vi "QMdiSubWindow.vi"(5 "parent":refnum<class "QWidget.lvclass">, 8 "Error In":errorcluster, 11 "Post-Bundled Subclass":refnum<class "QMdiSubWindow.lvclass">) -> (0 "Error Out":errorcluster, 3 "New QMdiSubWindow":refnum<class "QMdiSubWindow.lvclass">)   [LabVIEW 2014, in "QMdiSubWindow.lvclass"]
doc: "LabVIEW-specific documentation is not yet available. See <b>https://doc.qt.io/qt-5/qmdisubwindow.html#QMdiSubWindow</b>"
uses:
  QMdiSubWindow.lvclass
  QWidget/QWidget.lvclass
  LQ Core/LQCoreEngine/_Internal/LQIdentity Registry Action.ctl
  LQ Core/LQIdentity/LQIdentity.lvclass/LQIdentity.ctl
  LQ Core/LQCoreEngine/LQCoreEngine.lvclass
  LQ Core/LQ Core.lvlib
  LQ Core/LQIdentity/LQIdentity.lvclass
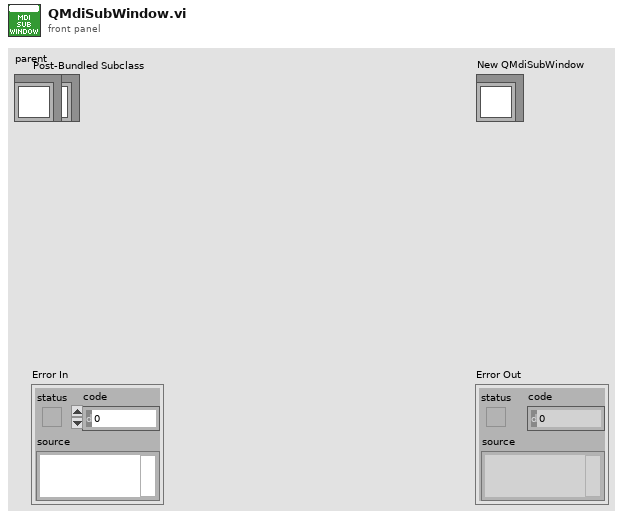
[diagram p1: front panel]
types:
  T1 = typedef "LQ Core.lvlib/LQCoreEngine.lvclass/LQIdentity Registry Action.ctl" = enum16{"Init", "Register LQIdentity", "Get LQIdentity Info", "Deregister LQIdentity"}
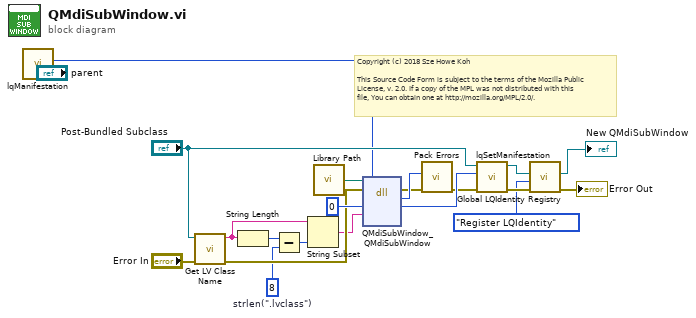
[diagram p0: block diagram]
diagram:
  w6 = 8  # strlen(".lvclass")
  # "Copyright (c) 2018 Sze Howe Koh\n\nThis Source Code Form is subject to the terms of the Mozilla Public\nLicense, v. 2.0. If a copy of the MPL was not distributed with this\nfile, You can obtain one at http://mozilla.org/MPL/2.0/."
  n1 = call "lqManifestation.vi"("LQIdentity in"="parent") -> ("Manifestation"=w1:u64)  [unwired: 9 in, 1 out]
  n2 = call <vilib>:"Get LV Class Name.vi"("error in (no error)"="Error In", "object"="Post-Bundled Subclass") -> ("error out"=w8:errorcluster, "class name"=w4:string)  [unwired: 8 in]
  n3 = String Length(string=w4) -> (length=w7:i32)
  n4 = Subtract(x=w7, y=w6) -> (x-y=w5:i32)
  n5 = String Subset(string=w4, length (rest)=w5) -> (substring=w3:string)  [unwired: 1 in]
  n6 = call "Library Path.vi"() -> ("Library Path"=w19:path)
  n7 = dll-call lib="?" fn="QMdiSubWindow_QMdiSubWindow"(path in=w19, error in=w8, "_retVal"=u64 0 ("_instance"), "_className"=w3, "parent"=w1) -> (error out=w17:errorcluster, w18:i32, "_retVal"=w20:u64)  [unwired: 3 in, 1 out]
  n8 = call "Pack Errors.vi"("Error In"=w17, "Error Code"=w18) -> ("Error Out"=w16:errorcluster)  [unwired: 9 in]
  n9 = call "lqSetManifestation.vi"("Error In"=w16, "Manifestation"=w20, "LQIdentity in"="Post-Bundled Subclass") -> ("Error Out"=w14:errorcluster, "LQIdentity out"=w15:refnum<class "QMdiSubWindow.lvclass">)  [unwired: 7 in]
  n10 = call "Global LQIdentity Registry.vi"("Error In"=w14, "Registry Action"=LQIdentity_Registry_Action."Register LQIdentity", "LQIdentity Info In"=w15) -> ("Error Out"=→"Error Out":errorcluster, "LQIdentity Info Out"=→"New QMdiSubWindow":refnum<class "QMdiSubWindow.lvclass">)  [unwired: 7 in]
